vi "EOD Write.vi"(0 "file path (use dialog)":path, 1 "EODDataInput":T1(array[cluster]) {"Nchar" format="%.0x"}) -> (7 "refnum out":refnum<file>, 10 "error out":errorcluster)   [LabVIEW 2014]
panel:
  # "MSU EFish Lab EOD Write File VI"
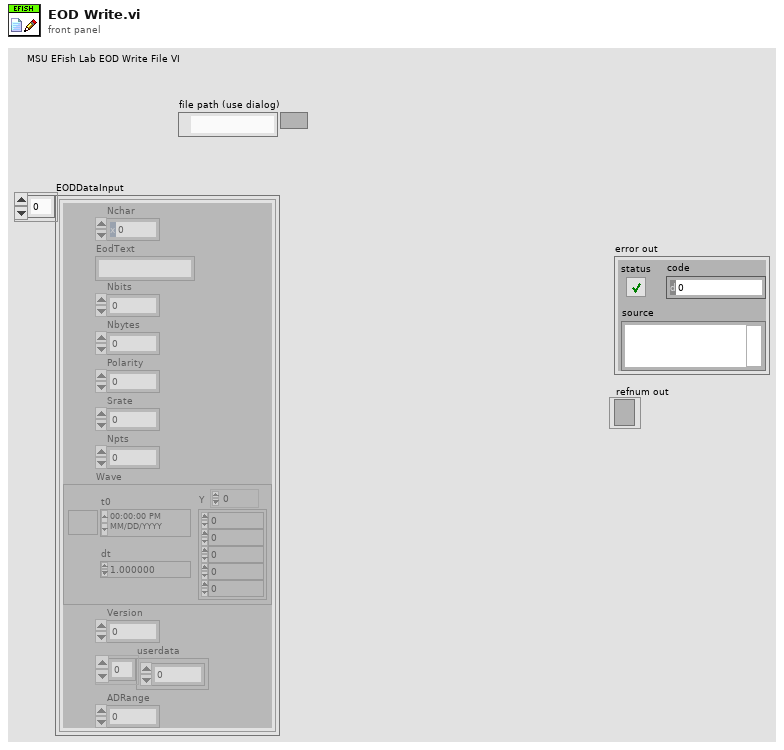
[diagram p1: front panel]
types:
  T1 = cluster{"Nchar":u8, "EodText":string, "Nbits":i32, "Nbytes":i32, "Polarity":i32, "Srate":i32, "Npts":i32, "Wave":waveform(dbl), "Version":i32, "userdata":dbl[], "ADRange":dbl}[]
  T2 = enum16{"open", "replace", "create", "open or create", "replace or create", "replace or create with confirmation"}
  T3 = enum16{"big-endian, network order", "native, host order", "little-endian"}
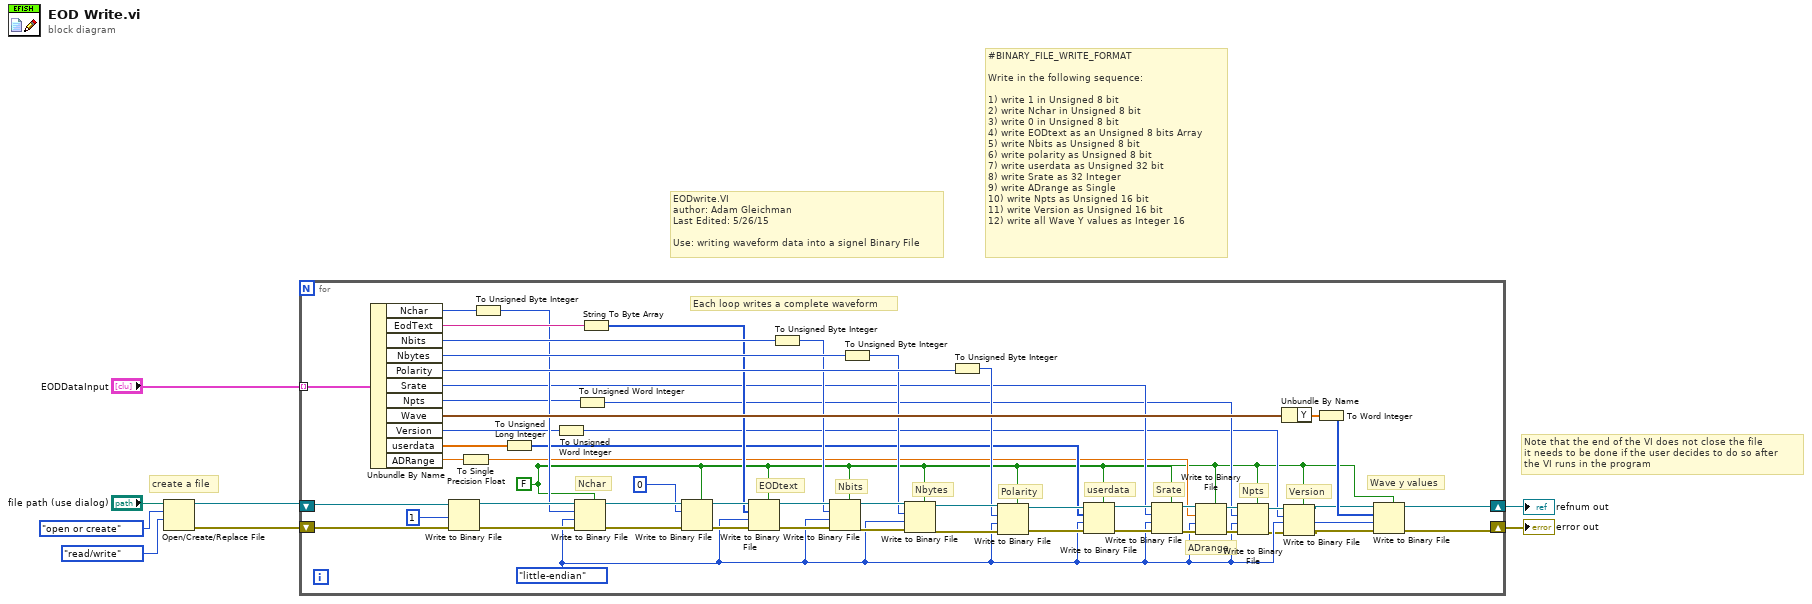
[diagram p0: block diagram]
diagram:
  # "Note that the end of the VI does not close the file\nit needs to be done if the user decides to do so after\nthe VI runs in the program"
  # "EODwrite.VI\nauthor: Adam Gleichman\nLast Edited: 5/26/15\n\nUse: writing waveform data into a signel Binary File"
  # "#BINARY_FILE_WRITE_FORMAT\n\nWrite in the following sequence:\n\n1) write 1 in Unsigned 8 bit\n2) write Nchar in Unsigned 8 bit\n3) write 0 in Unsigned 8 bit\n4) write EODtext as an Unsigned 8 bits Array\n5) write Nbits as Unsigned 8 bit\n6) write polarity as Unsigned 8 bit\n7) write userdata as Unsigned 32 bit\n8) write Srate as 32 Integer\n9) write ADrange as Single\n10) write Npts as Unsigned 16 bit\n11) write Version as Unsigned 16 bit\n12) write all Wave Y values as Integer 16"
  # "create a file"
  n1 = Open/Create/Replace File(file path (use dialog)="file path (use dialog)", operation (0:open)=T2."open or create", access (0:read/write)=enum16{"read/write", "read-only", "write-only"}."read/write") -> (refnum out=w6:refnum<file>, error out=w5:errorcluster)  [unwired: 3 in, 1 out]
  n2 = for {
    tunnel: "EODDataInput" -> [w63] mode=indexing
    shift-right: [w42] -> w4
    shift-left: w6 -> [w10]
    shift-right: [w41] -> w3
    shift-left: w5 -> [w9]
    w11 = FALSE
    w20 = T3."little-endian" ("byte order (0:big-endian, network order)")
    # "Each loop writes a complete waveform"
    # "Version"
    # "Npts"
    # "Wave y values"
    # "ADrange"
    # "Srate"
    # "userdata"
    # "Polarity"
    # "Nbytes"
    # "Nchar"
    # "Nbits"
    # "EODtext"
    n3 = Unbundle By Name(w63) -> ("Nchar"=w62:u8, "EodText"=w61:string, "Nbits"=w58:i32, "Nbytes"=w53:i32, "Polarity"=w52:i32, "Srate"=w27:i32, "Npts"=w21:i32, "Wave"=w45:waveform(dbl), "Version"=w13:i32, "userdata"=w49:dbl[], "ADRange"=w46:dbl)
    n4 = Write to Binary File(file (use dialog)=w10, data=u8 1, error in=w9) -> (refnum out=w34:refnum<file>, error out=w35:errorcluster)  [unwired: 3 in, 1 out]
    n5 = To Single Precision Float(number=w46) -> (single precision float=w18:sgl)
    n6 = To Unsigned Byte Integer(number=w62) -> (unsigned 8bit integer=w32:u8)
    n7 = To Unsigned Long Integer(number=w49) -> (unsigned 32bit integer=w26:u32[])
    n8 = To Unsigned Word Integer(number=w13) -> (unsigned 16bit integer=w12:u16)
    n9 = Write to Binary File(file (use dialog)=w34, data=w32, error in=w35, 5:w11, 9:w20) -> (refnum out=w40:refnum<file>, error out=w39:errorcluster)  [unwired: 1 in, 1 out]
    n10 = To Unsigned Word Integer(number=w21) -> (unsigned 16bit integer=w19:u16)
    n11 = String To Byte Array(string=w61) -> (unsigned byte array=w31:u8[])
    n12 = Write to Binary File(file (use dialog)=w40, data=u8 0, error in=w39, 5:w11) -> (refnum out=w38:refnum<file>, error out=w37:errorcluster)  [unwired: 2 in, 1 out]
    n13 = Write to Binary File(file (use dialog)=w38, data=w31, error in=w37, 5:w11, 9:w20) -> (refnum out=w60:refnum<file>, error out=w59:errorcluster)  [unwired: 1 in, 1 out]
    n14 = To Unsigned Byte Integer(number=w58) -> (unsigned 8bit integer=w30:u8)
    n15 = Write to Binary File(file (use dialog)=w60, data=w30, error in=w59, 5:w11, 9:w20) -> (refnum out=w57:refnum<file>, error out=w56:errorcluster)  [unwired: 1 in, 1 out]
    n16 = To Unsigned Byte Integer(number=w53) -> (unsigned 8bit integer=w29:u8)
    n17 = Write to Binary File(file (use dialog)=w57, data=w29, error in=w56, 5:w11, 9:w20) -> (refnum out=w55:refnum<file>, error out=w54:errorcluster)  [unwired: 1 in, 1 out]
    n18 = To Unsigned Byte Integer(number=w52) -> (unsigned 8bit integer=w28:u8)
    n19 = Write to Binary File(file (use dialog)=w55, data=w28, error in=w54, 5:w11, 9:w20) -> (refnum out=w51:refnum<file>, error out=w50:errorcluster)  [unwired: 1 in, 1 out]
    n20 = Write to Binary File(file (use dialog)=w51, data=w26, error in=w50, 5:w11, 9:w20) -> (refnum out=w48:refnum<file>, error out=w47:errorcluster)  [unwired: 1 in, 1 out]
    n21 = Write to Binary File(file (use dialog)=w48, data=w27, error in=w47, 5:w11, 9:w20) -> (refnum out=w25:refnum<file>, error out=w24:errorcluster)  [unwired: 1 in, 1 out]
    n22 = Write to Binary File(file (use dialog)=w25, data=w18, error in=w24, 5:w11, 9:w20) -> (refnum out=w23:refnum<file>, error out=w22:errorcluster)  [unwired: 1 in, 1 out]
    n23 = Write to Binary File(file (use dialog)=w23, data=w19, error in=w22, 5:w11, 9:w20) -> (refnum out=w14:refnum<file>, error out=w15:errorcluster)  [unwired: 1 in, 1 out]
    n24 = Unbundle By Name(w45) -> ("Y"=w44:dbl[])
    n25 = Write to Binary File(file (use dialog)=w14, data=w12, error in=w15, 5:w11) -> (refnum out=w17:refnum<file>, error out=w16:errorcluster)  [unwired: 2 in, 1 out]
    n26 = To Word Integer(number=w44) -> (16bit integer=w43:i16[])
    n27 = Write to Binary File(file (use dialog)=w17, data=w43, error in=w16, 5:w11, 9:w20) -> (refnum out=w42:refnum<file>, error out=w41:errorcluster)  [unwired: 1 in, 1 out]
  }
  "refnum out" <- w4
  "error out" <- w3
